vi "Get Pos Data.vi"(11 "AttMap":map{string, string}(c390)) -> (2 "FP Position":T1, 3 "Position":T1)   [LabVIEW 2025]
uses:
  <vilib>/Utility/miscctls.llb/LVPointTypeDef.ctl
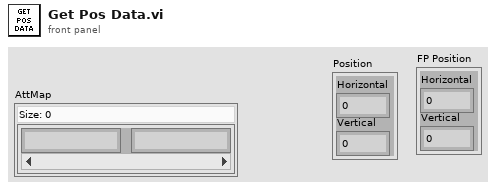
[diagram p1: front panel]
types:
  T1 = typedef "LVPointTypeDef.ctl" = cluster{"Horizontal":i16, "Vertical":i16}
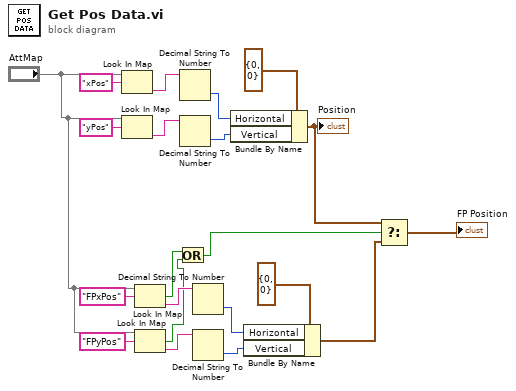
[diagram p0: block diagram]
diagram:
  n1 = Look In Map(map="AttMap", key="xPos") -> (value=w17:string)  [unwired: 1 in, 1 out]
  n2 = Look In Map(map="AttMap", key="yPos") -> (value=w18:string)  [unwired: 1 in, 1 out]
  n3 = Look In Map(map="AttMap", key="FPxPos") -> (key not found?=w6:bool, value=w12:string)  [unwired: 1 in]
  n4 = Look In Map(map="AttMap", key="FPyPos") -> (key not found?=w5:bool, value=w11:string)  [unwired: 1 in]
  n5 = Or(x=w6, y=w5) -> (x .or. y?=w3:bool)
  n6 = Decimal String To Number(string=w17) -> (number=w20:i32)  [unwired: 2 in, 1 out]
  n7 = Decimal String To Number(string=w18) -> (number=w21:i32)  [unwired: 2 in, 1 out]
  n8 = Decimal String To Number(string=w12) -> (number=w9:i32)  [unwired: 2 in, 1 out]
  n9 = Decimal String To Number(string=w11) -> (number=w8:i32)  [unwired: 2 in, 1 out]
  n10 = Bundle By Name(cluster=T1 {"Horizontal"=0, "Vertical"=0} ("location"), "Horizontal"=w20, "Vertical"=w21) -> (w2:T1)
  "Position" <- w2
  n11 = Bundle By Name(cluster=T1 {"Horizontal"=0, "Vertical"=0} ("location"), "Horizontal"=w9, "Vertical"=w8) -> (w4:T1)
  n12 = Select(t=w2, s=w3, f=w4) -> (s? t:f=→"FP Position":T1)
